vi "Pic Overlay Box.vi"(6 "Line":T1={"Width"=1, "Style"=enum."Solid"}, 8 "error in (no error)":errorcluster, 9 "Color":cluster{"Border Color":u32, "Fill Color":u32}={"Border Color"=16740207, "Fill Color"=16740207}, 10 "Rectangle":T2, 11 "Picture in":picture) -> (0 "error out":errorcluster, 3 "Picture out":picture)   [LabVIEW 2018, in "Picture Process.lvclass"]
uses:
  Picture Process.lvclass
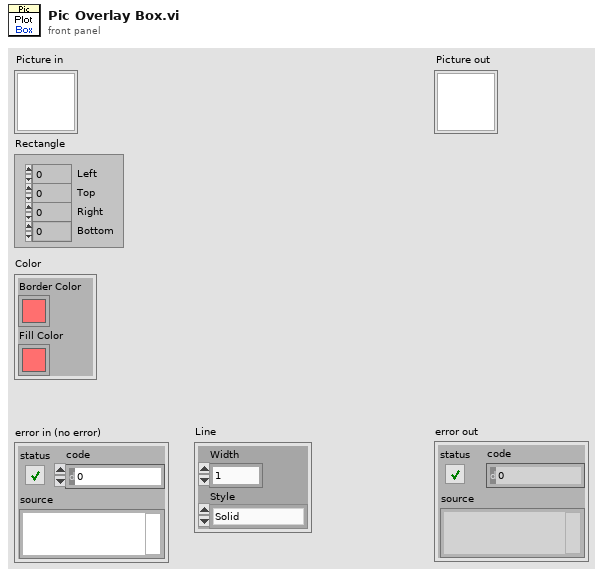
[diagram p1: front panel]
types:
  T1 = cluster{"Width":i16, "Style":enum32{"Solid", "Dash", "Dot", "DashDot", "DashDotDot"}}
  T2 = cluster{"Left":i32, "Top":i32, "Right":i32, "Bottom":i32}
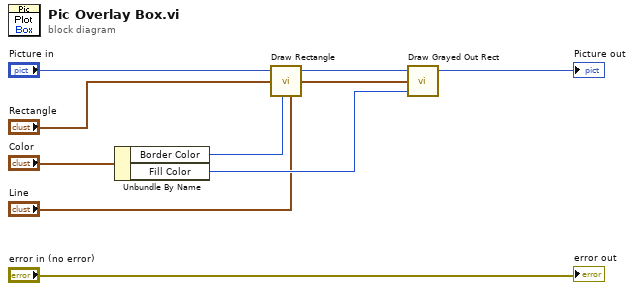
[diagram p0: block diagram]
diagram:
  n1 = Unbundle By Name("Color") -> ("Border Color"=w4:u32, "Fill Color"=w3:u32)
  n2 = call <vilib>:"Draw Rectangle.vi"("picture"="Picture in", "rect"="Rectangle", "color(black)"=w4, "pen"="Line") -> ("new picture"=w7:picture)  [unwired: 5 in]
  n3 = call <vilib>:"Draw Grayed Out Rect.vi"("color(black)"=w3, "rect"="Rectangle", "picture"=w7) -> ("new picture"=→"Picture out":picture)  [unwired: 2 in]
  "error out" <- "error in (no error)"
